vi "GetCompressionLevel.vi"(8 "Error In":errorcluster, 11 "reference in":refnum<class "CompressionDecorator.lvclass">) -> (0 "Error Out":errorcluster, 2 "Return(INT32)":i32, 3 "reference in":refnum<class "CompressionDecorator.lvclass">)   [LabVIEW 2020, in "CompressionDecorator.lvclass"]
uses:
  CompressionDecorator.lvclass
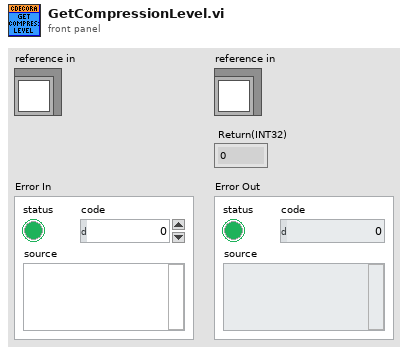
[diagram p1: front panel]
types:
  T1 = typedef "CompressionDecorator.lvclass/ObjectAttributes.ctl" = cluster{"CompLevel":i32}
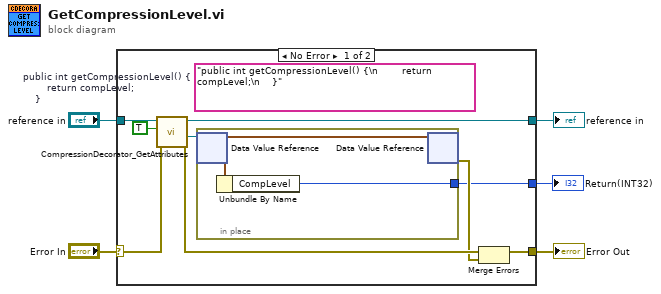
[diagram p0: block diagram]
diagram:
  n1 = case shown="No Error" "Error In" {
    selector: "Error In" -> [w13 w18]
    tunnel: [w12 w18] -> w4
    tunnel: [w11 w17] -> w2
    tunnel: "reference in" -> [w14 w17]
    tunnel: [w7 _] -> w1
    frame No Error {
      (unwired) "public int getCompressionLevel() {\n        return compLevel;\n    }"  # public int getCompressionLevel() {         return compLevel;     }
      n2 = call "CompressionDecorator_GetAttributes.vi"("error in (no error)"=w13, "OnlyGetDvrReference(False)"=TRUE, "reference in"=w14) -> ("error out"=w9:errorcluster, "DataRef"=w10:refnum<data-value>, "reference out"=w11:refnum<class "CompressionDecorator.lvclass">)  [unwired: 5 in, 1 out]
      n3 = in-place {
        in-place-border: [w16] -> w7
        n4 = in-place-dvr #1(w10) -> (w15:T1)  [unwired: 1 out]
        n5 = Unbundle By Name(w15) -> ("CompLevel"=w16:i32)
        n6 = in-place-dvr #1(w15) -> (w8:errorcluster)  [unwired: 1 out]
      }
      n7 = Merge Errors(w9, w8) -> (w12:errorcluster)
    }
    frame Error {
    }
  }
  "Error Out" <- w4
  "reference in" <- w2
  "Return(INT32)" <- w1
